vi "controller_total_cycle.vi"() -> ()   [LabVIEW 2026]
uses:
  C:/Program Files (x86)/Control/SC3U.dll
  Program Files (x86)/Control/SC3U.dll
panel:
  in  "Save To File":bool
  in  "Move Selected Down":bool=TRUE
  in  "Move Selected Up":bool=TRUE
  in  "Delete Selected Position":bool=TRUE
  in  "Save Current Position":enum16{"Add New", "Overwrite Selected"}(ring)
  in  "Saved Positions":i32(listbox) caption="Select to Change"
  in  "Go To Selected Position":bool=TRUE
  in  "Stage COM":u8=7
  in  "Arduino Digital \nOutput Channel":u8=13
  in  "Arduino COM":refnum<visa-resource-name>
  in  "Number of Cycles":i32=1
  out "Current Z":dbl
  out "Current Y":dbl
  out "Current X":dbl
  in  "?":bool
  in  "Stage Com Close":bool
  in  "SC3U":refnum<k24>(container)
  in  "Run Sequence":bool=TRUE
  in  "Save Current Position":bool=TRUE caption="Save"
  in  "Time Between Cycles (s)":dbl=1.0
  # "Set Connections"
  # "Set Duration"
  # "Saved Positions"
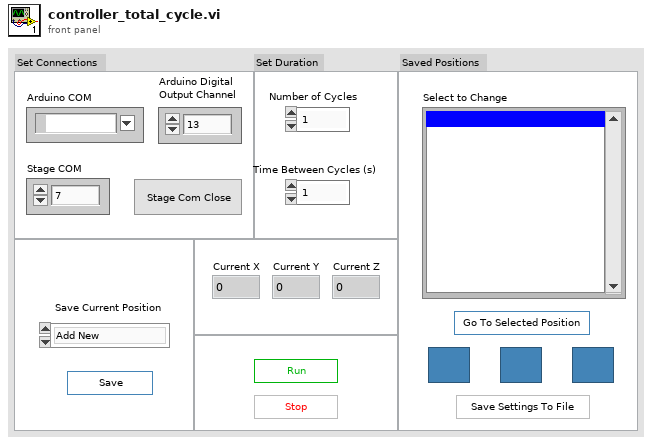
[diagram p1: front panel]
types:
  T1 = cluster{"GetCurrentPosition":dbl, "GetCurrentPosition":dbl, "GetCurrentPosition":dbl}
  T2 = cluster{"GetCurrentPosition":dbl, "GetCurrentPosition":dbl, "GetCurrentPosition":dbl}[]
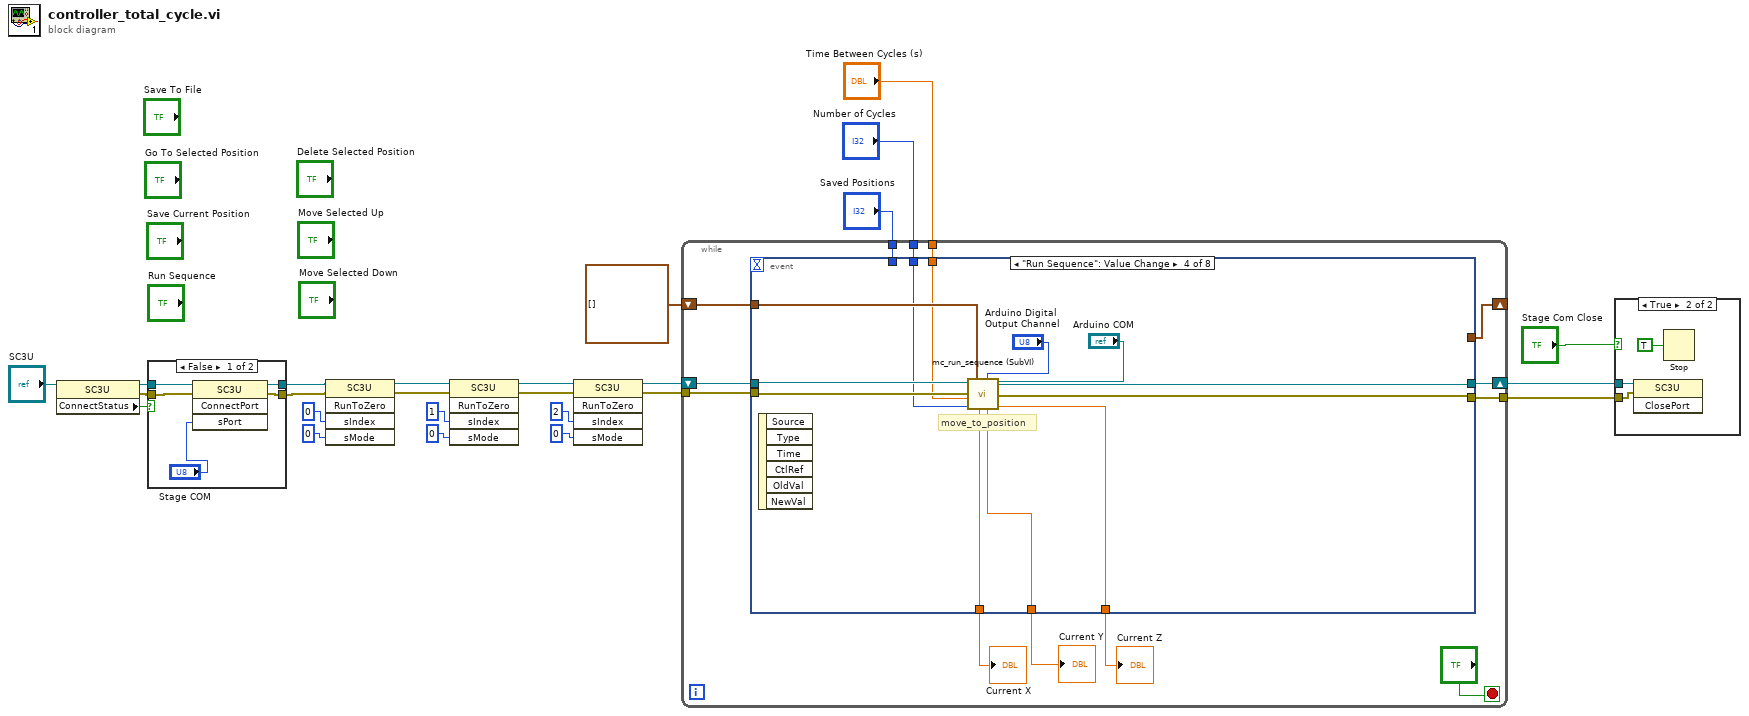
[diagram p0: block diagram]
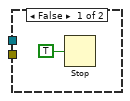
[diagram p2: hidden frame]
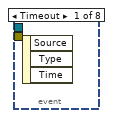
[diagram p4: hidden frame]
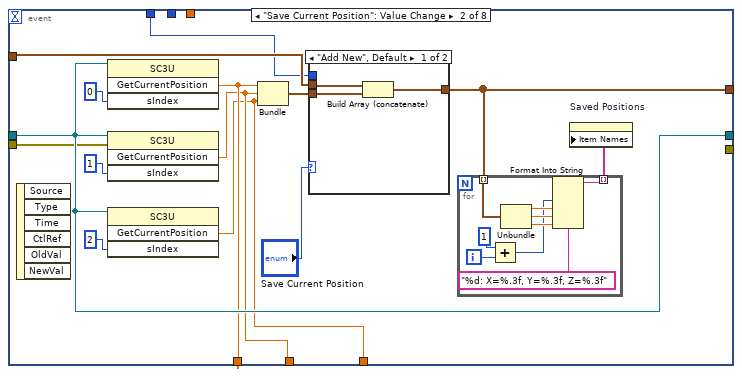
[diagram p5: hidden frame]
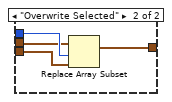
[diagram p6: hidden frame]
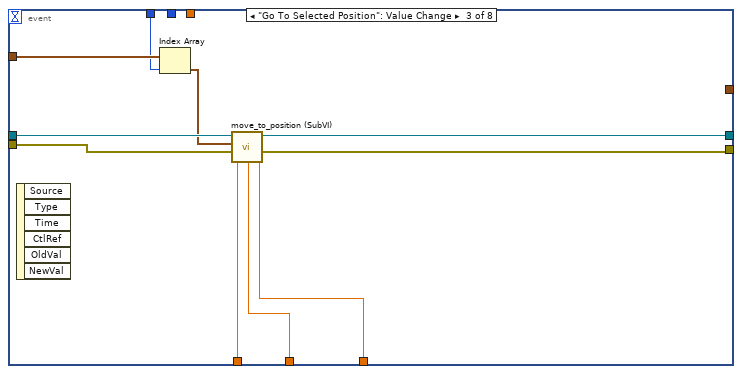
[diagram p7: hidden frame]
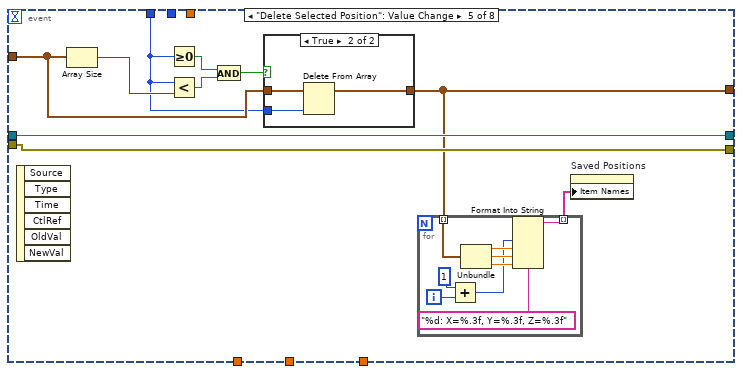
[diagram p8: hidden frame]
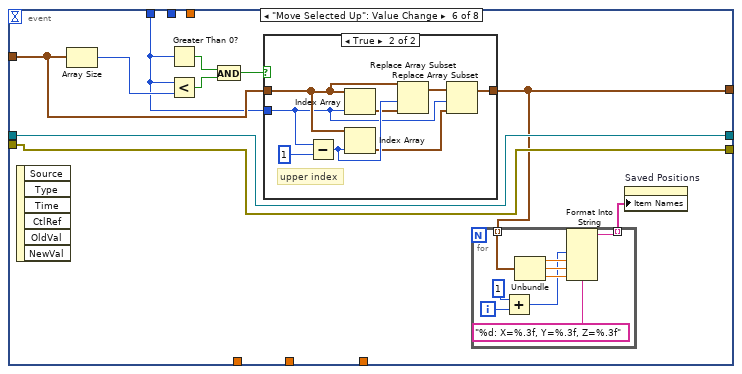
[diagram p10: hidden frame]
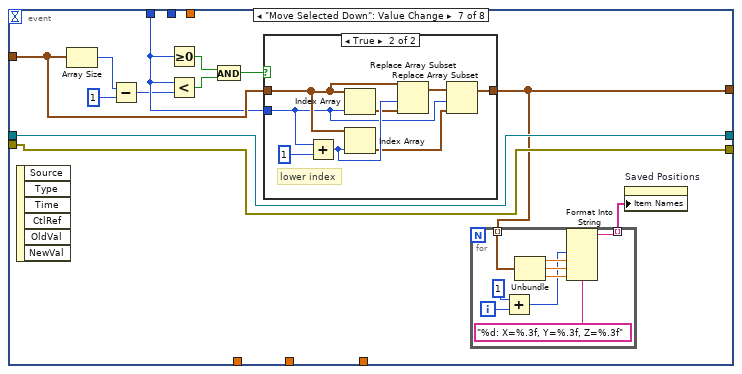
[diagram p12: hidden frame]
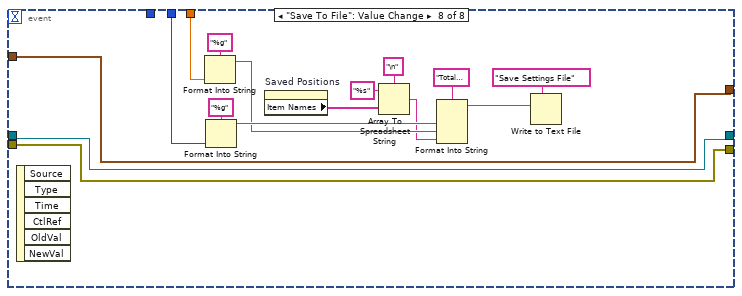
[diagram p14: hidden frame]
diagram:
  n1 = property class="SC3U"(reference="SC3U") -> (reference out=w24:refnum<k24>, error out=w19:errorcluster, "ConnectStatus"=w23:bool)  [unwired: 1 in]
  n2 = case shown="False" w23 {
    tunnel: w24 -> [w30 w32]
    tunnel: [w29 w32] -> w5
    tunnel: [w28 w31] -> w4
    tunnel: w19 -> [w27 w31]
    frame False {
      n3 = invoke class="SC3U" method="ConnectPort"(reference=w30, error in=w27, "sPort"="Stage COM") -> (reference out=w29:refnum<k24>, error out=w28:errorcluster)  [unwired: 1 in, 2 out]
    }
    frame True {
    }
  }
  n4 = invoke class="SC3U" method="RunToZero"(reference=w5, error in=w4, "sIndex"=i16 0, "sMode"=i16 0) -> (reference out=w17:refnum<k24>, error out=w14:errorcluster)  [unwired: 1 in, 3 out]
  n5 = invoke class="SC3U" method="RunToZero"(reference=w17, error in=w14, "sIndex"=i16 1, "sMode"=i16 0) -> (reference out=w16:refnum<k24>, error out=w15:errorcluster)  [unwired: 1 in, 3 out]
  n6 = invoke class="SC3U" method="RunToZero"(reference=w16, error in=w15, "sIndex"=i16 2, "sMode"=i16 0) -> (reference out=w6:refnum<k24>, error out=w7:errorcluster)  [unwired: 1 in, 3 out]
  n7 = while {
    shift-right: [w45] -> _
    shift-left: cluster{dbl, dbl, dbl}[] [] -> [w43]
    shift-right: [w42] -> w20
    shift-left: w6 -> [w44]
    tunnel: w7 -> [w41]
    tunnel: [w40] -> w18
    tunnel: "Saved Positions" -> [w35]
    tunnel: "Number of Cycles" -> [w34]
    tunnel: "Time Between Cycles (s)" -> [w33]
    stop <- "?" stop-if-true
    n8 = event shown="[3] \"Run Sequence\": Value Change" {
      selector: _ -> [_ _ _ _ _ _ _ _]
      dyn-events: _ -> [_ _ _ _ _ _ _ _]
      timeout: _ -> [_ _ _ _ _ _ _ _]
      tunnel: [_ w48 _ _ w99 w121 w152 w194] -> w45
      tunnel: [_ w56 w82 w93 w107 w122 w153 w182] -> w42
      tunnel: w44 -> [_ w56 w84 w96 w107 w122 w153 w182]
      tunnel: w43 -> [_ w47 w85 w97 w101 w126 w157 w194]
      tunnel: w41 -> [_ w55 w81 w95 w106 w123 w154 w183]
      tunnel: [_ _ w80 w94 w106 w123 w154 w183] -> w40
      tunnel: [_ w53 w79 w92 _ _ _ _] -> w38
      tunnel: [_ w52 w78 w86 _ _ _ _] -> w37
      tunnel: [_ w51 w77 w91 _ _ _ _] -> w36
      tunnel: w35 -> [_ w46 w76 _ w100 w125 w156 _]
      tunnel: w34 -> [_ _ _ w87 _ _ _ w192]
      tunnel: w33 -> [_ _ _ w88 _ _ _ w193]
      event Timeout {
        n9 = event-data() -> ()  [unwired: 1 in, 3 out]
      }
      event "Save Current Position": Value Change {
        n10 = event-data() -> ()  [unwired: 1 in, 6 out]
        n11 = invoke class="SC3U" method="GetCurrentPosition"(reference=w56, "sIndex"=i16 0) -> ("GetCurrentPosition"=w53:dbl)  [unwired: 2 in, 3 out]
        n12 = invoke class="SC3U" method="GetCurrentPosition"(reference=w56, error in=w55, "sIndex"=i16 1) -> ("GetCurrentPosition"=w52:dbl)  [unwired: 1 in, 3 out]
        n13 = invoke class="SC3U" method="GetCurrentPosition"(reference=w56, "sIndex"=i16 2) -> ("GetCurrentPosition"=w51:dbl)  [unwired: 2 in, 3 out]
        n14 = Bundle("GetCurrentPosition"=w53, "GetCurrentPosition"=w52, "GetCurrentPosition"=w51) -> (w49:T1)  [unwired: 1 in]
        n15 = case shown="\"Add New\", Default" "Save Current Position" {
          tunnel: w47 -> [w70 w73]
          tunnel: w49 -> [w69 w74]
          tunnel: [w71 w72] -> w48
          tunnel: w46 -> [_ w75]
          frame "Add New", Default {
            n16 = Build Array (concatenate)(w70, w69) -> (w71:T2)
          }
          frame "Overwrite Selected" {
            n17 = Replace Array Subset(array=w73, new element=w74, index=w75) -> (w72:cluster{dbl, dbl, dbl}[])
          }
        }
        n18 = for {
          tunnel: w48 -> [w68] mode=indexing
          tunnel: [w60] -> w54 mode=indexing
          i -> [w63]
          n19 = Add(x=1 ("y"), y=w63) -> (x+y=w61:i32)
          n20 = Unbundle(w68) -> ("GetCurrentPosition"=w64:dbl, "GetCurrentPosition"=w65:dbl, "GetCurrentPosition"=w66:dbl)
          n21 = Format Into String(format string="%d: X=%.3f, Y=%.3f, Z=%.3f", w61, w64, w65, w66) -> (resulting string=w60:string)  [unwired: 2 in, 1 out]
        }
        n22 = property on="Saved Positions" class="LstBox (strict)"("Item Names"=w54) -> ()  [unwired: 2 in, 2 out]
      }
      event "Go To Selected Position": Value Change {
        n23 = event-data() -> ()  [unwired: 1 in, 6 out]
        n24 = Index Array(array=w85, index=w76) -> (element=w83:cluster{dbl, dbl, dbl})
        n25 = call "move_to_position (SubVI).vi"("error in (no error)"=w81, "Cluster"=w83, ".NET Refnum in"=w84) -> ("Current Z"=w77:dbl, "error out"=w80:errorcluster, ".NET Refnum out"=w82:refnum<k24>, "Current Y"=w78:dbl, "Current X"=w79:dbl)  [unwired: 4 in]
      }
      event "Run Sequence": Value Change {
        # "move_to_position"
        n26 = event-data() -> ()  [unwired: 1 in, 6 out]
        n27 = call "mc_run_sequence (SubVI).vi"("Basler COM"="Arduino COM", "Arduino Digital \nOutput Channel"="Arduino Digital \nOutput Channel", "Array"=w97, "Number of Cycles"=w87, "Time Between Cycles (s)"=w88, "error in (no error)"=w95, ".NET Refnum in"=w96) -> ("Current Z"=w91:dbl, "error out"=w94:errorcluster, ".NET Refnum out"=w93:refnum<k24>, "Current Y"=w86:dbl, "Current X"=w92:dbl)
      }
      event "Delete Selected Position": Value Change {
        n28 = event-data() -> ()  [unwired: 1 in, 6 out]
        n29 = Array Size(array=w101) -> (size(s)=w105:i32)
        n30 = Greater Or Equal To 0?(x=w100) -> (x >= 0?=w103:bool)
        n31 = Less?(x=w100, y=w105) -> (x < y?=w104:bool)
        n32 = And(x=w103, y=w104) -> (x .and. y?=w102:bool)
        n33 = case shown="True" w102 {
          tunnel: w101 -> [w117 w120]
          tunnel: w100 -> [_ w119]
          tunnel: [w117 w118] -> w99
          frame False {
          }
          frame True {
            n34 = Delete From Array(array=w120, index=w119) -> (array with subset deleted=w118:cluster{dbl, dbl, dbl}[])  [unwired: 1 in, 1 out]
          }
        }
        n35 = for {
          tunnel: w99 -> [w116] mode=indexing
          tunnel: [w108] -> w98 mode=indexing
          i -> [w111]
          n36 = Add(x=1 ("y"), y=w111) -> (x+y=w109:i32)
          n37 = Unbundle(w116) -> (w112:dbl, w113:dbl, w114:dbl)
          n38 = Format Into String(format string="%d: X=%.3f, Y=%.3f, Z=%.3f", w109, w112, w113, w114) -> (resulting string=w108:string)  [unwired: 2 in, 1 out]
        }
        n39 = property on="Saved Positions" class="LstBox (strict)"("Item Names"=w98) -> ()  [unwired: 2 in, 2 out]
      }
      event "Move Selected Up": Value Change {
        n40 = event-data() -> ()  [unwired: 1 in, 6 out]
        n41 = Array Size(array=w126) -> (size(s)=w130:i32)
        n42 = Greater Than 0?(x=w125) -> (x > 0?=w128:bool)
        n43 = Less?(x=w125, y=w130) -> (x < y?=w129:bool)
        n44 = And(x=w128, y=w129) -> (x .and. y?=w127:bool)
        n45 = case shown="True" w127 {
          tunnel: w126 -> [w140 w145]
          tunnel: w125 -> [_ w142]
          tunnel: [w140 w141] -> w121
          frame False {
          }
          frame True {
            # "upper index"
            n46 = Subtract(x=w142, y=1) -> (x-y=w147:i32)
            n47 = Index Array(array=w145, index=w142) -> (element=w146:cluster{dbl, dbl, dbl})
            n48 = Index Array(array=w145, index=w147) -> (element=w144:cluster{dbl, dbl, dbl})
            n49 = Replace Array Subset(array=w145, new element=w146, index=w147) -> (w143:cluster{dbl, dbl, dbl}[])
            n50 = Replace Array Subset(array=w143, new element=w144, index=w142) -> (w141:cluster{dbl, dbl, dbl}[])
          }
        }
        n51 = for {
          tunnel: w121 -> [w139] mode=indexing
          tunnel: [w131] -> w124 mode=indexing
          i -> [w134]
          n52 = Add(x=1 ("y"), y=w134) -> (x+y=w132:i32)
          n53 = Unbundle(w139) -> (w135:dbl, w136:dbl, w137:dbl)
          n54 = Format Into String(format string="%d: X=%.3f, Y=%.3f, Z=%.3f", w132, w135, w136, w137) -> (resulting string=w131:string)  [unwired: 2 in, 1 out]
        }
        n55 = property on="Saved Positions" class="LstBox (strict)"("Item Names"=w124) -> ()  [unwired: 2 in, 2 out]
      }
      event "Move Selected Down": Value Change {
        n56 = event-data() -> ()  [unwired: 1 in, 6 out]
        n57 = Array Size(array=w157) -> (size(s)=w151:i32)
        n58 = Subtract(x=w151, y=1) -> (x-y=w150:i32)
        n59 = Greater Or Equal To 0?(x=w156) -> (x >= 0?=w159:bool)
        n60 = Less?(x=w156, y=w150) -> (x < y?=w160:bool)
        n61 = And(x=w159, y=w160) -> (x .and. y?=w158:bool)
        n62 = case shown="True" w158 {
          tunnel: w157 -> [w170 w175]
          tunnel: w156 -> [_ w172]
          tunnel: [w170 w171] -> w152
          frame False {
          }
          frame True {
            # "lower index"
            n63 = Add(x=w172, y=1) -> (x+y=w177:i32)
            n64 = Index Array(array=w175, index=w172) -> (element=w176:cluster{dbl, dbl, dbl})
            n65 = Index Array(array=w175, index=w177) -> (element=w174:cluster{dbl, dbl, dbl})
            n66 = Replace Array Subset(array=w175, new element=w176, index=w177) -> (w173:cluster{dbl, dbl, dbl}[])
            n67 = Replace Array Subset(array=w173, new element=w174, index=w172) -> (w171:cluster{dbl, dbl, dbl}[])
          }
        }
        n68 = for {
          tunnel: w152 -> [w169] mode=indexing
          tunnel: [w161] -> w155 mode=indexing
          i -> [w164]
          n69 = Add(x=1 ("y"), y=w164) -> (x+y=w162:i32)
          n70 = Unbundle(w169) -> (w165:dbl, w166:dbl, w167:dbl)
          n71 = Format Into String(format string="%d: X=%.3f, Y=%.3f, Z=%.3f", w162, w165, w166, w167) -> (resulting string=w161:string)  [unwired: 2 in, 1 out]
        }
        n72 = property on="Saved Positions" class="LstBox (strict)"("Item Names"=w155) -> ()  [unwired: 2 in, 2 out]
      }
      event "Save To File": Value Change {
        n73 = event-data() -> ()  [unwired: 1 in, 6 out]
        n74 = Format Into String(format string="%g", w193) -> (resulting string=w185:string)  [unwired: 2 in, 1 out]
        n75 = Format Into String(format string="%g", w192) -> (resulting string=w186:string)  [unwired: 2 in, 1 out]
        n76 = property on="Saved Positions" class="LstBox (strict)"() -> ("Item Names"=w189:string[])  [unwired: 2 in, 2 out]
        n77 = Array To Spreadsheet String(delimiter (Tab)="\n", array=w189, 3:"%s" ("format string")) -> (spreadsheet string=w184:string)
        n78 = Format Into String(format string="Total Time: %s\\nTime Between Cycles: %s\\nSaved Positions:\\n%s", w186, w185, w184) -> (resulting string=w181:string)  [unwired: 2 in, 1 out]
        n79 = Write to Text File(prompt (Choose or enter file path)="Save Settings File", text=w181) -> ()  [unwired: 2 in, 3 out]
      }
    }
    "Current X" <- w38
    "Current Y" <- w37
    "Current Z" <- w36
  }
  n80 = case shown="True" "Stage Com Close" {
    tunnel: w20 -> [_ w198]
    tunnel: w18 -> [_ w196]
    frame False {
      n81 = Stop(stop? (T)=TRUE) -> ()
    }
    frame True {
      n82 = invoke class="SC3U" method="ClosePort"(reference=w198, error in=w196) -> ()  [unwired: 1 in, 3 out]
      n83 = Stop(stop? (T)=TRUE) -> ()
    }
  }
